vi "与副屏通信master.vi"() -> ()   [LabVIEW 2016, in "斯坦道多参数.lvlib"]
uses:
  <vilib>/NI/Modbus Library/API/Wrapper/Create TCP Master.vi
  <vilib>/NI/Modbus Library/API/master/Modbus Master.lvclass
  <vilib>/NI/Modbus Library/API/Wrapper/API Main.lvlib
  <vilib>/ptbypt/NI_PtbyPt.lvlib
panel:
  out "副屏启动命令":u16
  in  "停止 2":bool
  out "read values 2":u16[](array[numeric])
  in  "registers to write 2":u16[](array[numeric])
  out "error out 2":errorcluster caption="error out"
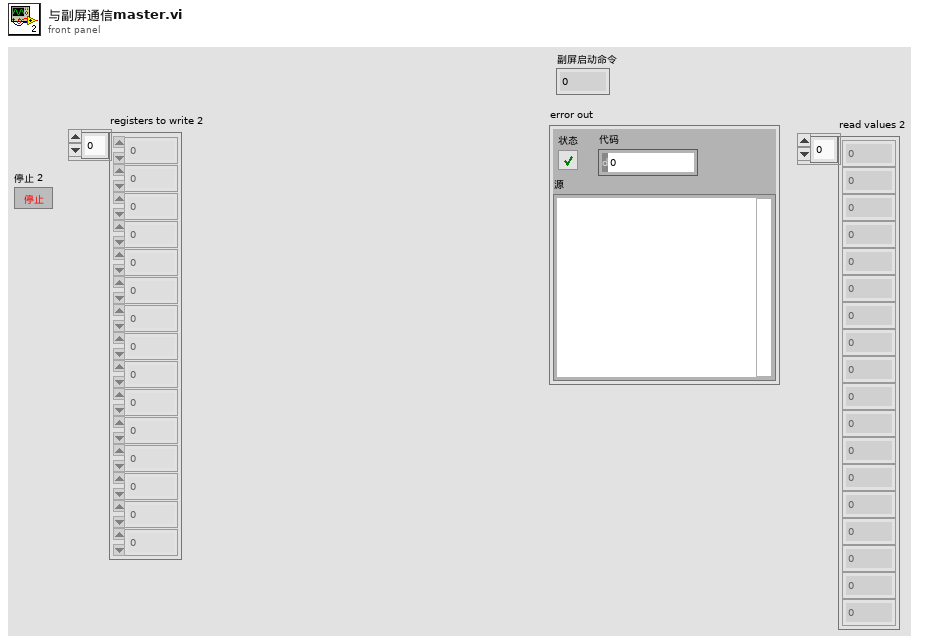
[diagram p1: front panel]
types:
  T1 = cluster{"数据保存间隔":dbl, "水温标样值":dbl, "pH标样值":dbl, "溶解氧标样值":dbl, "电导率标样值":dbl, "浊度标样值":dbl}
  T2 = cluster{"Boolean array[0]":bool, "Boolean array[1]":bool, "Boolean array[2]":bool, "Boolean array[3]":bool, "Boolean array[4]":bool, "Boolean array[5]":bool, "Boolean array[6]":bool}
  T3 = enum32{"Bad", "Idle", "Run top level", "Running"}
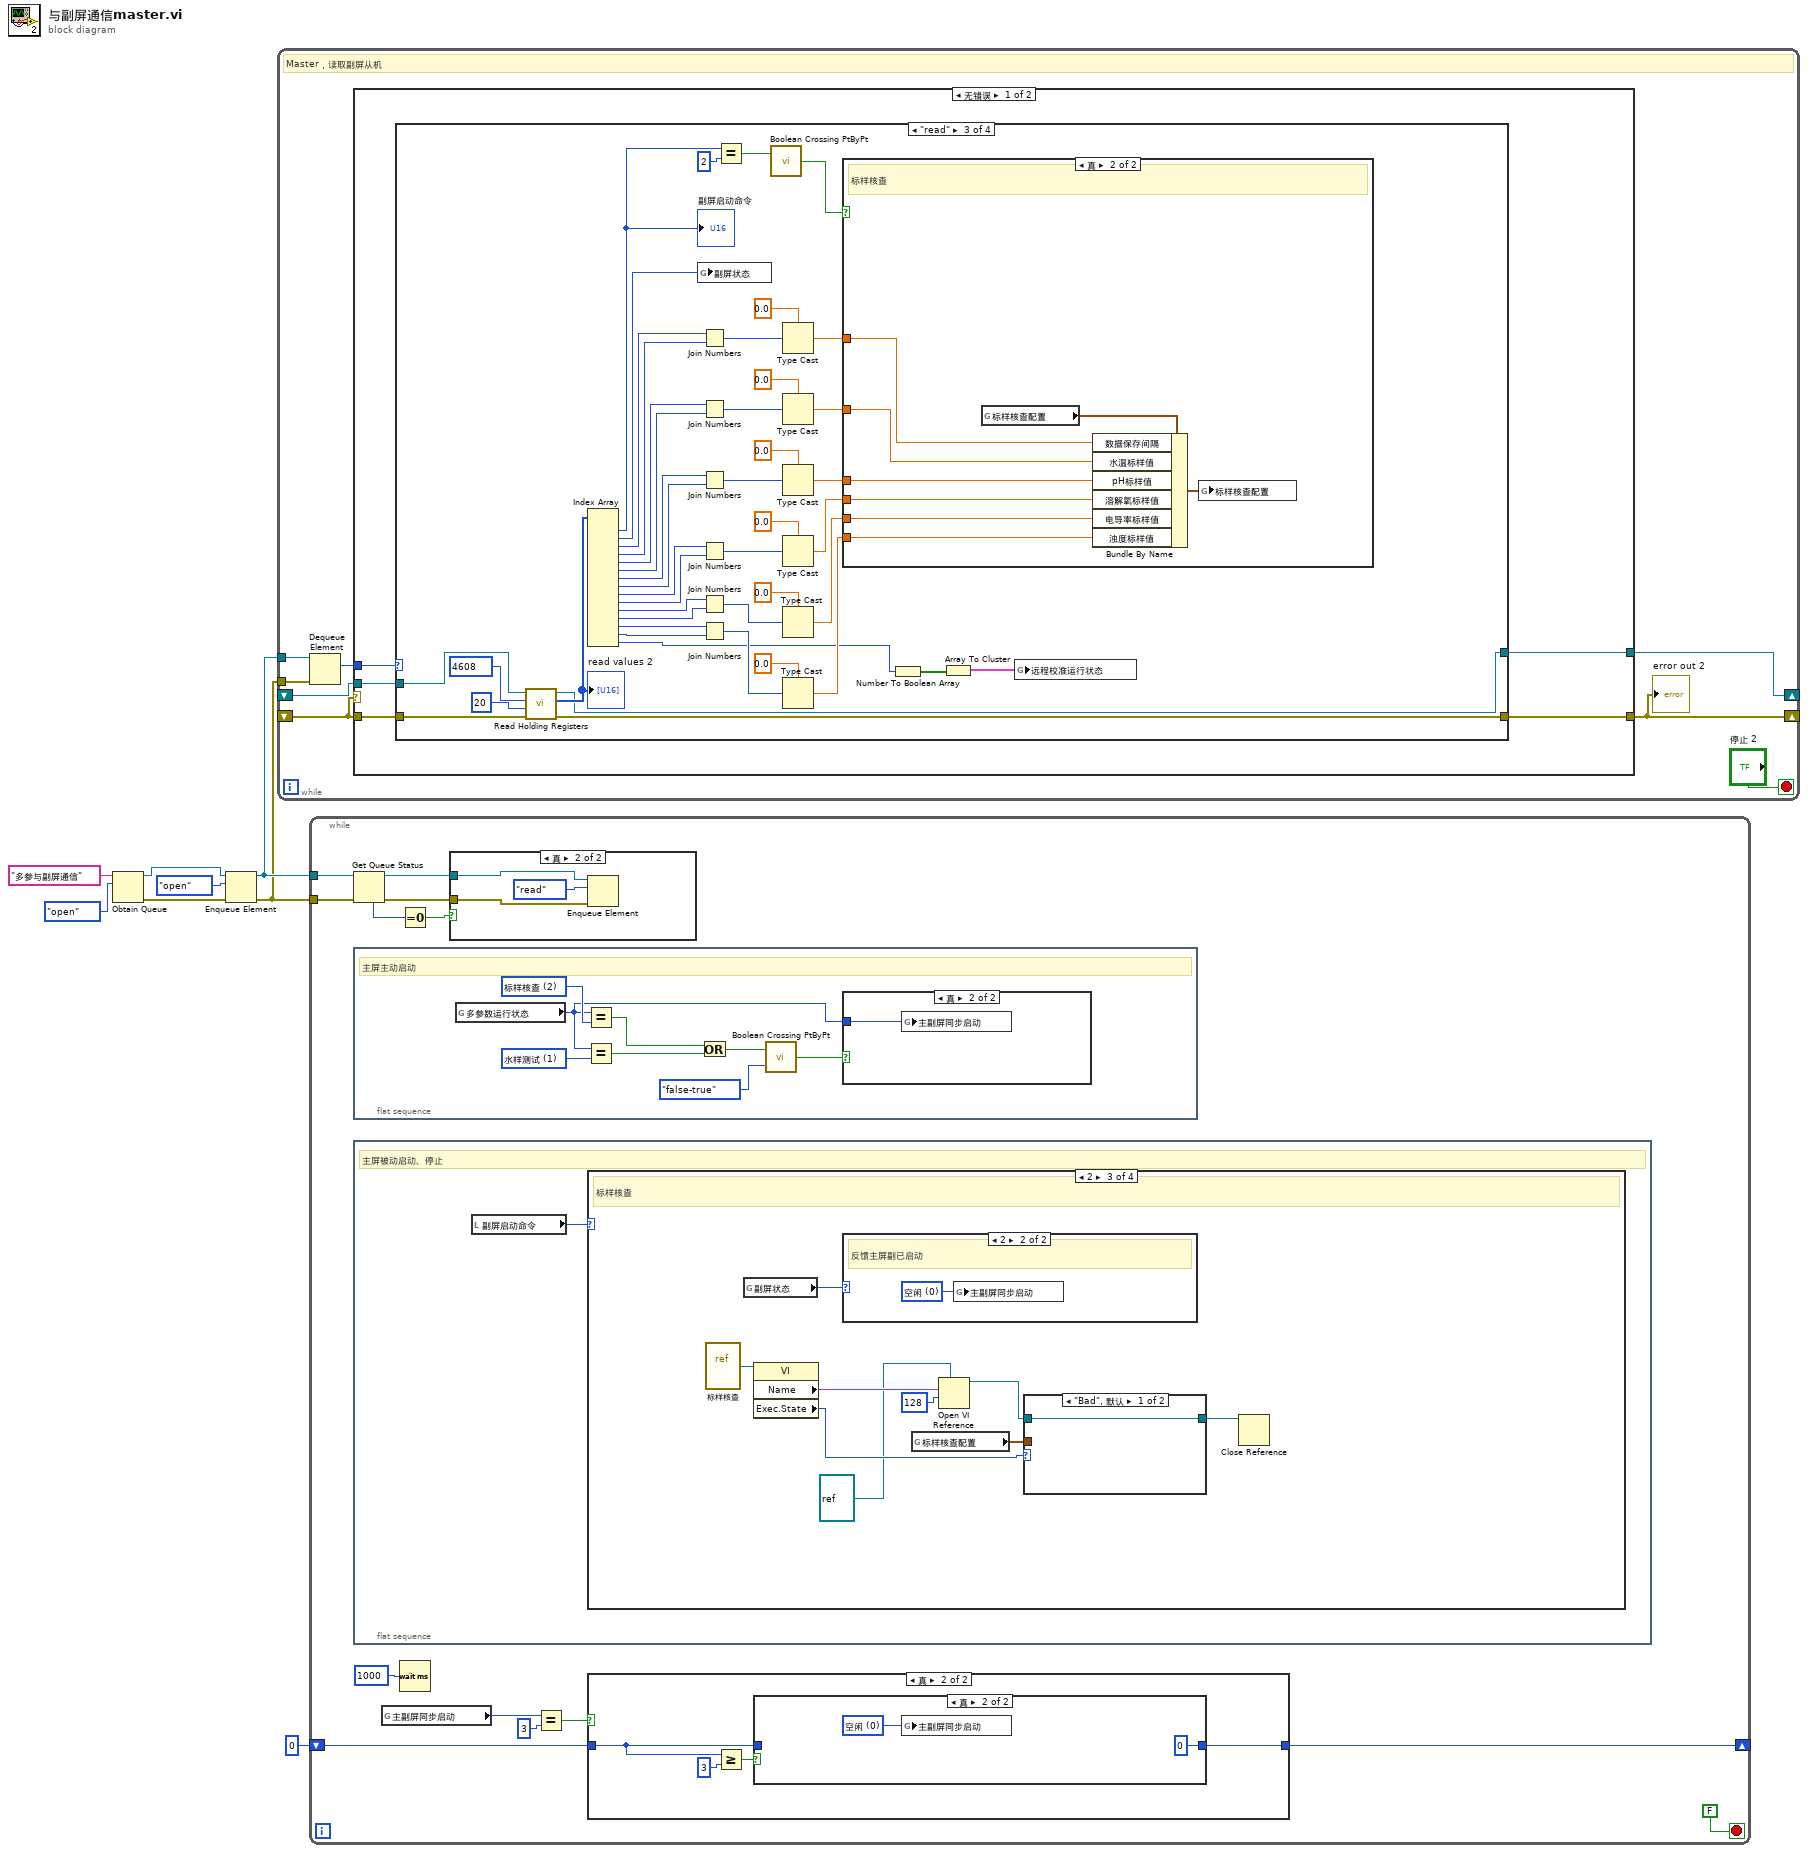
[diagram p0: block diagram]
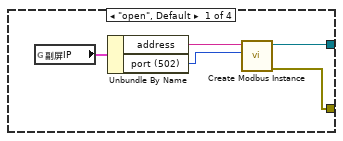
[diagram p2: hidden frame]
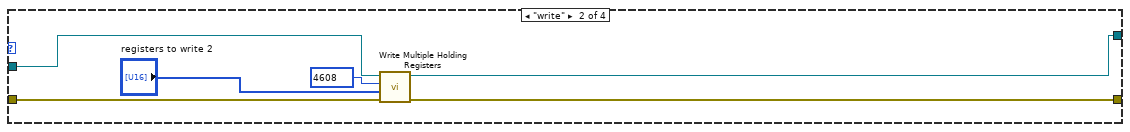
[diagram p3: hidden frame]
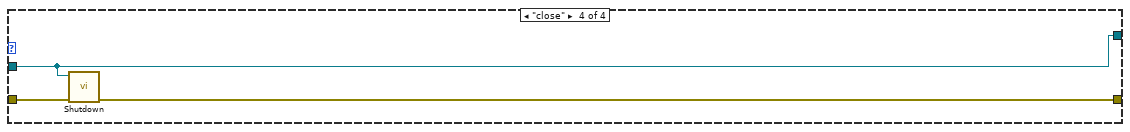
[diagram p5: hidden frame]
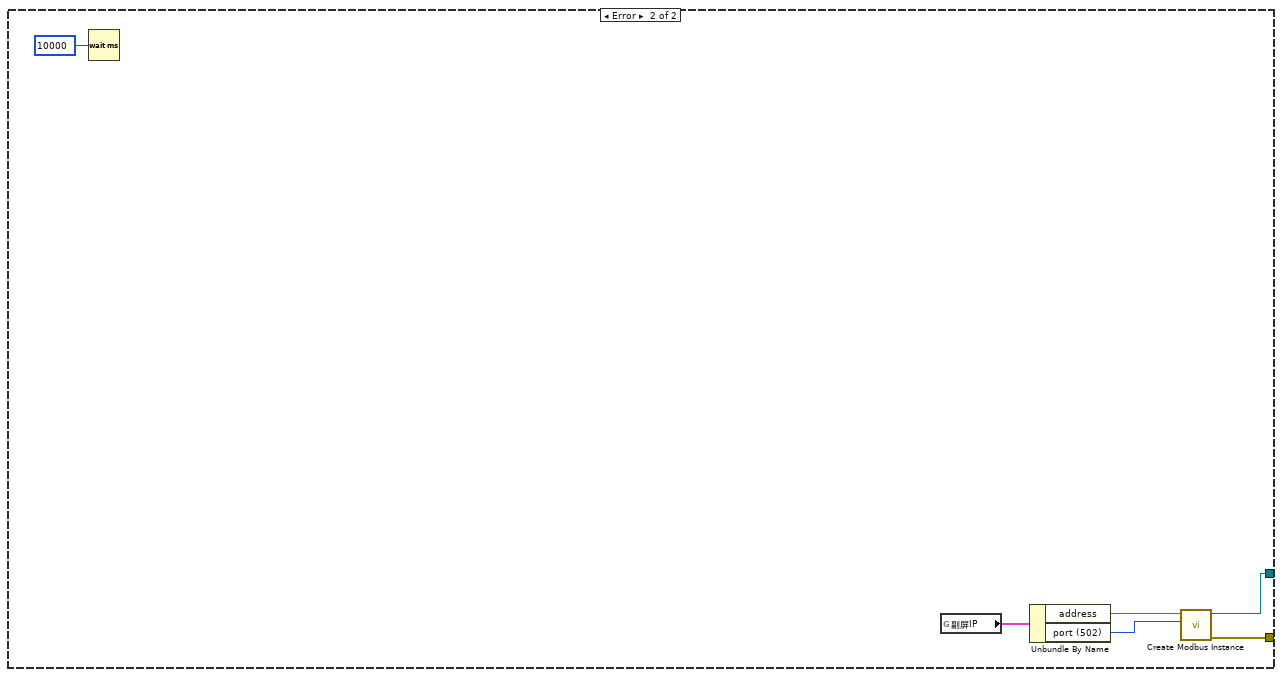
[diagram p6: hidden frame]
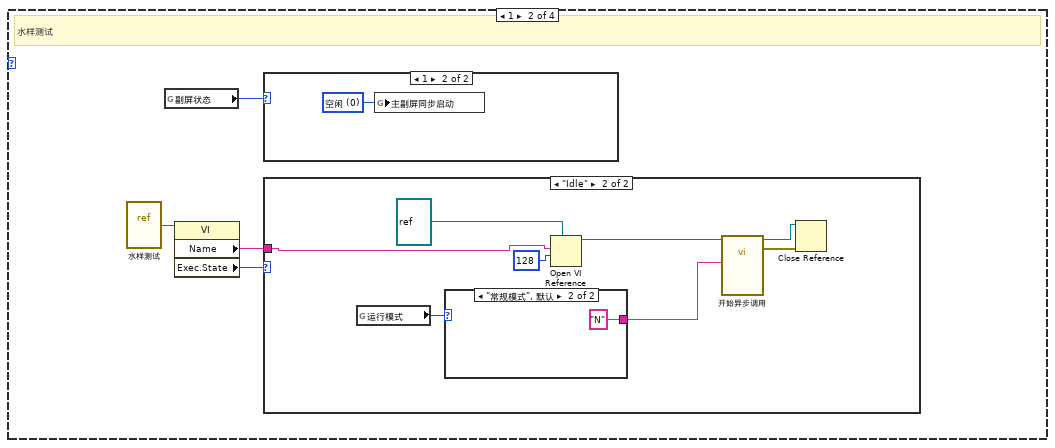
[diagram p8: hidden frame]
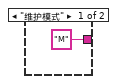
[diagram p11: hidden frame]
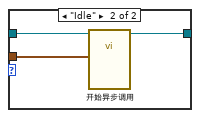
[diagram p13: hidden frame]
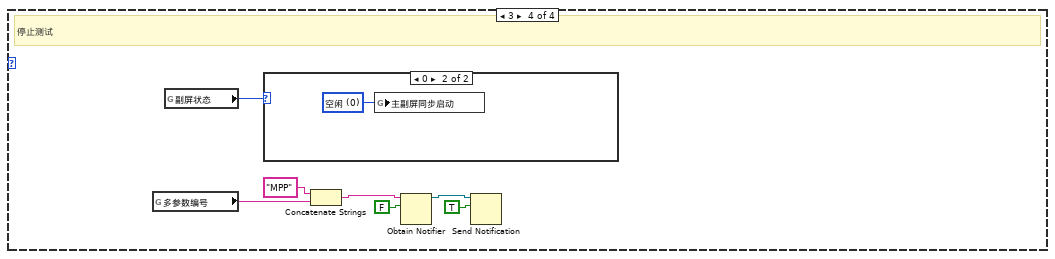
[diagram p14: hidden frame]
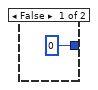
[diagram p16: hidden frame]
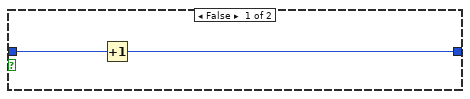
[diagram p17: hidden frame]
diagram:
  n1 = Obtain Queue(name (unnamed)="多参与副屏通信" ("名称（未命名）"), element data type=enum16{"open", "write", "read", "close"}."open") -> (queue out=w5:refnum<queue>, error out=w6:errorcluster)  [unwired: 3 in, 1 out]
  n2 = Enqueue Element(queue=w5, element=enum16{"open", "write", "read", "close"}."open", error in (no error)=w6) -> (queue out=w3:refnum<queue>, error out=w2:errorcluster)  [unwired: 1 in, 1 out]
  n3 = while {
    shift-right: [w13] -> _
    shift-left: _ -> [w15]
    shift-right: [w14] -> _
    shift-left: _ -> [w12]
    tunnel: w3 -> [w11]
    tunnel: w2 -> [w10]
    stop <- "停止 2" stop-if-true
    # "Master，读取副屏从机"
    n4 = Dequeue Element(queue=w11, error in (no error)=w10) -> (element=w9:enum16{"open", "write", "read", "close"})  [unwired: 1 in, 3 out]
    n5 = case shown="无错误" w12 {
      tunnel: w15 -> [w21 _]
      tunnel: w12 -> [w20 _]
      tunnel: [w19 w93] -> w14
      tunnel: [w18 w94] -> w13
      tunnel: w9 -> [w17 _]
      frame No Error {
        n6 = case shown="\"read\"" w17 {
          tunnel: w21 -> [_ w32 w39 w88]
          tunnel: w20 -> [_ w30 w38 w87]
          tunnel: [w25 w27 w36 w86] -> w19
          tunnel: [w26 w28 w37 w88] -> w18
          frame "open", Default {
            n7 = global read "多参数全局变量.vi" "副屏IP"() -> (w24:cluster{"address":string, "port (502)":u16})
            n8 = Unbundle By Name(w24) -> ("address"=w23:string, "port (502)"=w22:u16)
            n9 = call-poly <vilib>:"Create Modbus Instance.vi"("port (502)"=w22, "address"=w23) -> ("error out"=w25:errorcluster, "TCP master instance"=w26:refnum<class "Modbus Master.lvclass">)  [unwired: 8 in]
          }
          frame "write" {
            n10 = call-dynamic "Write Multiple Holding Registers.vi"("error in"=w30, "registers to write"="registers to write 2", "starting address"=u16 4608 ("write starting address"), "Modbus master in"=w32) -> ("error out"=w27:errorcluster, "Modbus master out"=w28:refnum<class "Modbus Master.lvclass">)  [unwired: 6 in]
          }
          frame "read" {
            n11 = call-dynamic "Read Holding Registers.vi"("error in"=w38, "number of inputs"=u16 20 ("read count"), "starting address"=u16 4608 ("write starting address"), "Modbus master in"=w39) -> ("error out"=w36:errorcluster, "register values"=w75:u16[], "Modbus master out"=w37:refnum<class "Modbus Master.lvclass">)  [unwired: 5 in]
            "read values 2" <- w75
            n12 = Index Array(array=w75) -> (element #1=w76:u16, element #2=w77:u16, element #3=w44:u16, element #4=w45:u16, element #5=w51:u16, element #6=w50:u16, element #7=w55:u16, element #8=w54:u16, element #9=w60:u16, element #10=w61:u16, element #11=w68:u16, element #12=w69:u16, element #13=w70:u16, element #14=w71:u16, element #15=w33:u16)  [unwired: 15 in]
            "副屏启动命令" <- w76
            n13 = global write "多参数全局变量.vi" "副屏状态"(w77) -> ()
            n14 = Join Numbers(hi=w44, lo=w45) -> ((hi.lo)=w43:u32)
            n15 = Join Numbers(hi=w51, lo=w50) -> ((hi.lo)=w48:u32)
            n16 = Join Numbers(hi=w55, lo=w54) -> ((hi.lo)=w53:u32)
            n17 = Join Numbers(hi=w60, lo=w61) -> ((hi.lo)=w58:u32)
            n18 = Join Numbers(hi=w68, lo=w69) -> ((hi.lo)=w63:u32)
            n19 = Join Numbers(hi=w70, lo=w71) -> ((hi.lo)=w65:u32)
            n20 = Equal?(x=w76, y=u16 2) -> (x = y?=w73:bool)
            n21 = call <vilib>:"Boolean Crossing PtByPt.vi"("input"=w73) -> ("crossing"=w74:bool)  [unwired: 2 in]
            n22 = Type Cast(type=sgl 0.0, x=w43) -> (*(type *) &x=w46:sgl)
            n23 = Type Cast(type=sgl 0.0, x=w48) -> (*(type *) &x=w49:sgl)
            n24 = Type Cast(type=sgl 0.0, x=w53) -> (*(type *) &x=w56:sgl)
            n25 = Type Cast(type=sgl 0.0, x=w58) -> (*(type *) &x=w59:sgl)
            n26 = Type Cast(type=sgl 0.0, x=w63) -> (*(type *) &x=w66:sgl)
            n27 = Type Cast(type=sgl 0.0, x=w65) -> (*(type *) &x=w67:sgl)
            n28 = case shown="真" w74 {
              tunnel: w46 -> [_ w83]
              tunnel: w49 -> [_ w82]
              tunnel: w56 -> [_ w81]
              tunnel: w59 -> [_ w80]
              tunnel: w66 -> [_ w79]
              tunnel: w67 -> [_ w78]
              frame False {
              }
              frame True {
                # "标样核查"
                n29 = global read "断电保存变量.vi" "标样核查配置"() -> (w85:T1)
                n30 = Bundle By Name(cluster=w85, "数据保存间隔"=w83, "水温标样值"=w82, "pH标样值"=w81, "溶解氧标样值"=w80, "电导率标样值"=w79, "浊度标样值"=w78) -> (w84:T1)
                n31 = global write "断电保存变量.vi" "标样核查配置"(w84) -> ()
              }
            }
            n32 = Number To Boolean Array(number=w33) -> (Boolean array=w35:bool[])
            n33 = Array To Cluster(array=w35) -> (cluster=w34:T2)
            n34 = global write "多参数全局变量.vi" "远程校准运行状态"(w34) -> ()
          }
          frame "close" {
            n35 = call-dynamic "Shutdown.vi"("error in"=w87, "Modbus master in"=w88) -> ("error out"=w86:errorcluster)  [unwired: 9 in]
          }
        }
      }
      frame Error {
        n36 = Wait (ms)(milliseconds to wait=u32 10000 ("等待时间（毫秒）")) -> ()  [unwired: 1 out]
        n37 = global read "多参数全局变量.vi" "副屏IP"() -> (w91:cluster{"address":string, "port (502)":u16})
        n38 = Unbundle By Name(w91) -> ("address"=w90:string, "port (502)"=w89:u16)
        n39 = call-poly <vilib>:"Create Modbus Instance.vi"("port (502)"=w89, "address"=w90) -> ("error out"=w93:errorcluster, "TCP master instance"=w94:refnum<class "Modbus Master.lvclass">)  [unwired: 8 in]
      }
    }
    "error out 2" <- w14
  }
  n40 = while {
    tunnel: w3 -> [w101]
    tunnel: w2 -> [w100]
    shift-right: [w95] -> _
    shift-left: u32 0 ("等待时间（毫秒）") -> [w96]
    stop <- FALSE stop-if-true
    n41 = Get Queue Status(queue=w101, error in (no error)=w100) -> (queue out=w103:refnum<queue>, error out=w104:errorcluster, # elements in queue=w102:i32)  [unwired: 1 in, 5 out]
    n42 = flat-sequence {
      frame #0 {
        w157 = u16 2 items=["空闲", "水样测试", "标样核查"] ("多参数运行状态")
        w160 = u16 1 items=["空闲", "水样测试", "标样核查"] ("多参数运行状态")
        # "主屏主动启动"
        n43 = global read "多参数全局变量.vi" "多参数运行状态"() -> (w156:u16)
        n44 = Equal?(x=w156, y=w157) -> (x = y?=w155:bool)
        n45 = Equal?(x=w156, y=w160) -> (x = y?=w161:bool)
        n46 = Or(x=w155, y=w161) -> (x .or. y?=w158:bool)
        n47 = call <vilib>:"Boolean Crossing PtByPt.vi"("direction"=enum16{"either", "false-true", "true-false"}."false-true", "input"=w158) -> ("crossing"=w159:bool)  [unwired: 1 in]
        n48 = case shown="真" w159 {
          tunnel: w156 -> [_ w163]
          frame False {
          }
          frame True {
            n49 = global write "多参数全局变量.vi" "主副屏同步启动"(w163) -> ()
          }
        }
      }
    }
    n50 = flat-sequence {
      frame #0 {
        # "主屏被动启动、停止"
        n51 = local read "副屏启动命令"() -> (w108:u16)
        n52 = case shown="2" w108 {
          frame 0, Default {
          }
          frame 1 {
            # "水样测试"
            n53 = vi-ref "水样测试.vi"() -> (w112:refnum<vi>)
            n54 = global read "多参数全局变量.vi" "副屏状态"() -> (w109:u16)
            n55 = property class="VI"(reference=w112) -> ("Name"=w110:string, "Exec.State"=w111:T3)  [unwired: 1 in, 2 out]
            n56 = case shown="1" w109 {
              frame 0, Default {
              }
              frame 1 {
                w113 = u16 0 items=["空闲", "水样测试", "标样核查", "停止"] ("主副屏同步启动")
                n57 = global write "多参数全局变量.vi" "主副屏同步启动"(w113) -> ()
              }
            }
            n58 = case shown="\"Idle\"" w111 {
              tunnel: w110 -> [_ w118]
              frame "Bad", Default {
              }
              frame "Idle" {
                n59 = global read "多参数全局变量.vi" "运行模式"() -> (w116:enum16{"维护模式", "常规模式", "应急模式", "质控模式"})
                n60 = case shown="\"常规模式\", 默认" w116 {
                  tunnel: ["M" ("数据标记表") "N" ("数据标记表")] -> w115
                  frame "维护模式" {
                  }
                  frame "常规模式", Default {
                  }
                }
                n61 = Open VI Reference(type specifier VI Refnum (for type only)=refnum<vi> refnum, vi path=w118, options=128 ("选项")) -> (vi reference=w119:refnum<vi>)  [unwired: 3 in, 1 out]
                n62 = call-by-ref "开始异步调用"(reference=w119, "数据标记表"=w115) -> (reference out=w120:refnum<vi>, error out=w121:errorcluster)  [unwired: 12 in]
                n63 = Close Reference(reference=w120, error in (no error)=w121) -> ()  [unwired: 1 out]
              }
            }
          }
          frame 2 {
            # "标样核查"
            n64 = vi-ref "标样核查.vi"() -> (w131:refnum<vi>)
            n65 = global read "多参数全局变量.vi" "副屏状态"() -> (w132:u16)
            n66 = property class="VI"(reference=w131) -> ("Name"=w127:string, "Exec.State"=w129:T3)  [unwired: 1 in, 2 out]
            n67 = case shown="2" w132 {
              frame 0, Default {
              }
              frame 2 {
                w133 = u16 0 items=["空闲", "水样测试", "标样核查", "停止"] ("主副屏同步启动")
                # "反馈主屏副已启动"
                n68 = global write "多参数全局变量.vi" "主副屏同步启动"(w133) -> ()
              }
            }
            n69 = global read "断电保存变量.vi" "标样核查配置"() -> (w125:T1)
            n70 = Open VI Reference(type specifier VI Refnum (for type only)=refnum<vi> refnum, vi path=w127, options=128 ("选项")) -> (vi reference=w126:refnum<vi>)  [unwired: 3 in, 1 out]
            n71 = case shown="\"Bad\", 默认" w129 {
              tunnel: [w134 w137] -> w130
              tunnel: w126 -> [w134 w136]
              tunnel: w125 -> [_ w135]
              frame "Bad", Default {
              }
              frame "Idle" {
                n72 = call-by-ref "开始异步调用"(reference=w136, "标样核查配置"=w135) -> (reference out=w137:refnum<vi>)  [unwired: 12 in, 1 out]
              }
            }
            n73 = Close Reference(reference=w130) -> ()  [unwired: 1 in, 1 out]
          }
          frame 3 {
            # "停止测试"
            n74 = global read "多参数全局变量.vi" "多参数编号"() -> (w141:string)
            n75 = global read "多参数全局变量.vi" "副屏状态"() -> (w138:u16)
            n76 = case shown="0" w138 {
              frame 1, Default {
              }
              frame 0 {
                w145 = u16 0 items=["空闲", "水样测试", "标样核查", "停止"] ("主副屏同步启动")
                n77 = global write "多参数全局变量.vi" "主副屏同步启动"(w145) -> ()
              }
            }
            n78 = Concatenate Strings("MPP" ("名称（未命名）"), w141) -> (w142:string)
            n79 = Obtain Notifier(name (unnamed)=w142, notification data type=FALSE) -> (notifier out=w139:refnum<notifier>)  [unwired: 2 in, 2 out]
            n80 = Send Notification(notification=TRUE ("通知"), notifier=w139) -> ()  [unwired: 1 in, 2 out]
          }
        }
      }
    }
    n81 = global read "多参数全局变量.vi" "主副屏同步启动"() -> (w99:u16)
    n82 = Equal To 0?(x=w102) -> (x = 0?=w105:bool)
    n83 = Wait (ms)(milliseconds to wait=u32 1000 ("等待时间（毫秒）")) -> ()  [unwired: 1 out]
    n84 = case shown="真" w105 {
      tunnel: w103 -> [_ w165]
      tunnel: w104 -> [_ w164]
      frame False {
      }
      frame True {
        n85 = Enqueue Element(queue=w165, element=enum16{"open", "write", "read", "close"}."read", error in (no error)=w164) -> ()  [unwired: 1 in, 3 out]
      }
    }
    n86 = Equal?(x=w99, y=u16 3) -> (x = y?=w97:bool)
    n87 = case shown="真" w97 {
      tunnel: w96 -> [_ w149]
      tunnel: [u32 0 w150] -> w95
      frame False {
      }
      frame True {
        n88 = Greater Or Equal?(x=w149, y=u32 3) -> (x >= y?=w147:bool)
        n89 = case shown="真" w147 {
          tunnel: [w152 u32 0] -> w150
          tunnel: w149 -> [w151 _]
          frame False {
            n90 = Increment(x=w151) -> (x+1=w152:u32)
          }
          frame True {
            w154 = u16 0 items=["空闲", "水样测试", "标样核查", "停止"] ("主副屏同步启动")
            n91 = global write "多参数全局变量.vi" "主副屏同步启动"(w154) -> ()
          }
        }
      }
    }
  }
